vi "Read All Digital Channels.vi"(7 "error in (no error)":errorcluster, 10 "VISA resource name":refnum<visa-resource-name>) -> (0 "error out":errorcluster, 2 "Digital Outputs":T1, 3 "VISA resource name out":refnum<visa-resource-name>)   [LabVIEW 2020, in "BDAQ-6104.lvlib"]
doc: "Read all digital input pins."
uses:
  <instrlib>/BDAQ-6104/BDAQ-6104.lvlib
panel:
  out "read buffer":string
  in  "DIO CLuster":T1
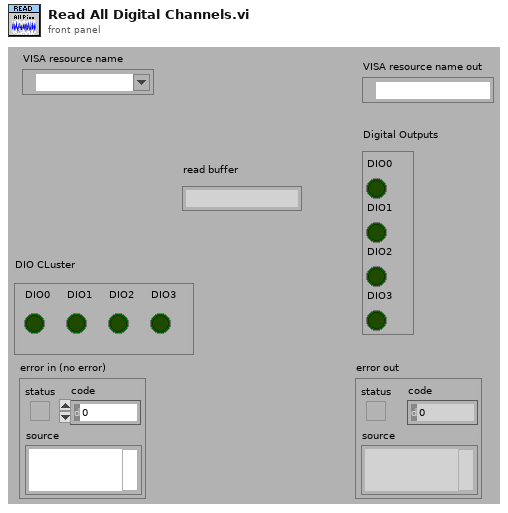
[diagram p1: front panel]
types:
  T1 = cluster{"DIO0":bool, "DIO1":bool, "DIO2":bool, "DIO3":bool}
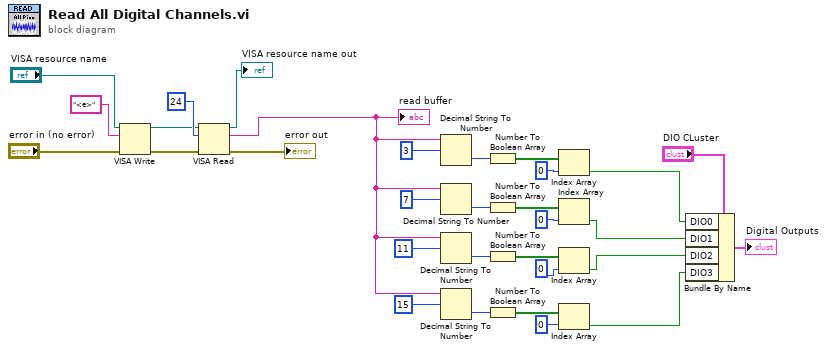
[diagram p0: block diagram]
diagram:
  n1 = VISA Write(VISA resource name="VISA resource name", write buffer="<e>" ("command"), error in (no error)="error in (no error)") -> (VISA resource name out=w25:refnum<visa-resource-name>, error out=w29:errorcluster)  [unwired: 1 out]
  n2 = VISA Read(VISA resource name=w25, byte count=u32 24, error in (no error)=w29) -> (VISA resource name out=→"VISA resource name out":refnum<visa-resource-name>, read buffer=w2:string, error out=→"error out":errorcluster)  [unwired: 1 out]
  "read buffer" <- w2
  n3 = Decimal String To Number(string=w2, offset=3) -> (number=w23:i32)  [unwired: 1 in, 1 out]
  n4 = Decimal String To Number(string=w2, offset=7) -> (number=w19:i32)  [unwired: 1 in, 1 out]
  n5 = Decimal String To Number(string=w2, offset=11) -> (number=w15:i32)  [unwired: 1 in, 1 out]
  n6 = Decimal String To Number(string=w2, offset=15) -> (number=w11:i32)  [unwired: 1 in, 1 out]
  n7 = Number To Boolean Array(number=w23) -> (Boolean array=w22:bool[])
  n8 = Number To Boolean Array(number=w19) -> (Boolean array=w18:bool[])
  n9 = Number To Boolean Array(number=w15) -> (Boolean array=w14:bool[])
  n10 = Number To Boolean Array(number=w11) -> (Boolean array=w10:bool[])
  n11 = Index Array(array=w22, index=0) -> (element=w8:bool)
  n12 = Index Array(array=w18, index=0) -> (element=w7:bool)
  n13 = Index Array(array=w14, index=0) -> (element=w6:bool)
  n14 = Index Array(array=w10, index=0) -> (element=w4:bool)
  n15 = Bundle By Name(cluster="DIO CLuster", "DIO0"=w8, "DIO1"=w7, "DIO2"=w6, "DIO3"=w4) -> (→"Digital Outputs":T1)
